vi "lab3.vi"() -> ()   [LabVIEW 2018]
uses:
  <vilib>/Utility/file.llb/Write Delimited Spreadsheet (DBL).vi
panel:
  out "unsigned byte array 2":u8[](array[numeric])
  out "Xincr":string
  out "Yoff":string
  out "Ymult":string
  out "error out 3":errorcluster
  in  "error in (no error) 4":errorcluster
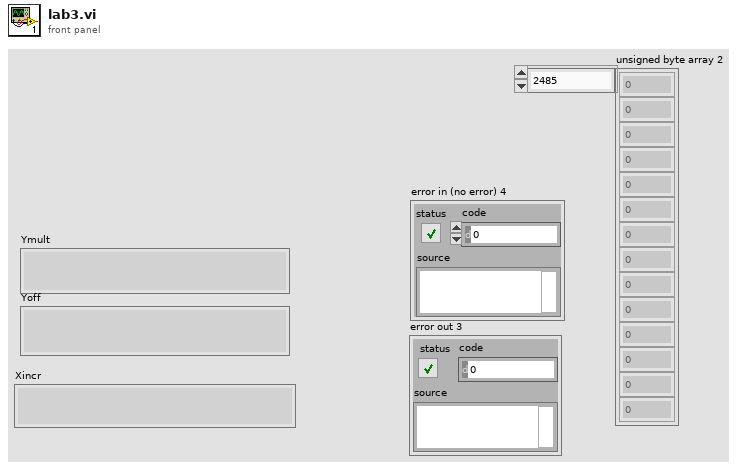
[diagram p1: front panel]
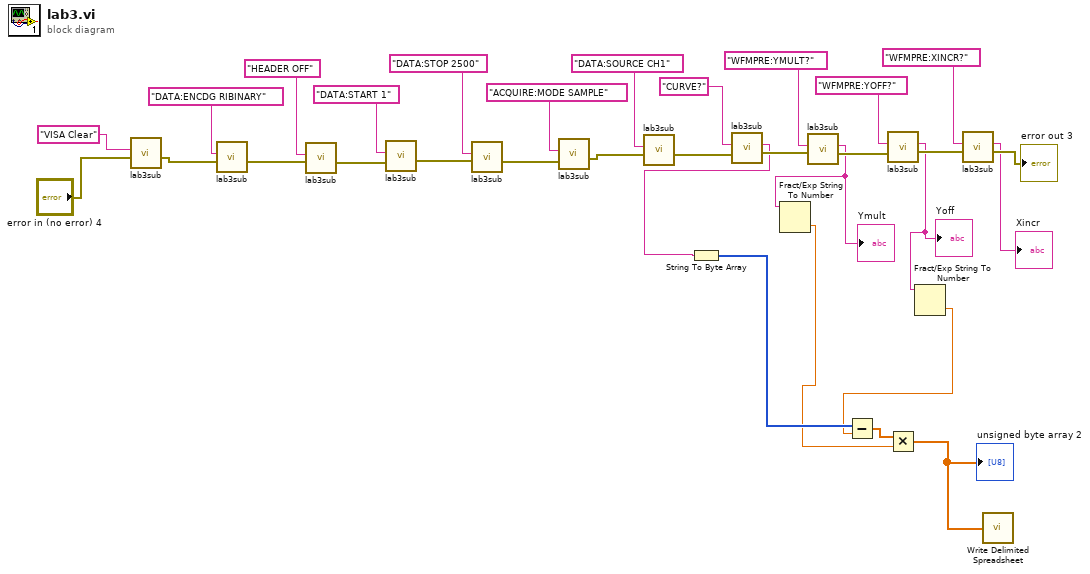
[diagram p0: block diagram]
diagram:
  n1 = call "lab3sub.vi"("error in (no error)"="error in (no error) 4", "write buffer"="VISA Clear") -> ("error out 2"=w21:errorcluster)  [unwired: 8 in, 1 out]
  n2 = call "lab3sub.vi"("error in (no error)"=w21, "write buffer"="DATA:ENCDG RIBINARY") -> ("error out 2"=w20:errorcluster)  [unwired: 8 in, 1 out]
  n3 = call "lab3sub.vi"("error in (no error)"=w20, "write buffer"="HEADER OFF") -> ("error out 2"=w19:errorcluster)  [unwired: 8 in, 1 out]
  n4 = call "lab3sub.vi"("error in (no error)"=w19, "write buffer"="DATA:START 1") -> ("error out 2"=w17:errorcluster)  [unwired: 8 in, 1 out]
  n5 = call "lab3sub.vi"("error in (no error)"=w17, "write buffer"="DATA:STOP 2500") -> ("error out 2"=w16:errorcluster)  [unwired: 8 in, 1 out]
  n6 = call "lab3sub.vi"("error in (no error)"=w16, "write buffer"="ACQUIRE:MODE SAMPLE") -> ("error out 2"=w15:errorcluster)  [unwired: 8 in, 1 out]
  n7 = call "lab3sub.vi"("error in (no error)"=w15, "write buffer"="DATA:SOURCE CH1") -> ("error out 2"=w14:errorcluster)  [unwired: 8 in, 1 out]
  n8 = call "lab3sub.vi"("error in (no error)"=w14, "write buffer"="CURVE?") -> ("error out 2"=w13:errorcluster, "read buffer"=w8:string)  [unwired: 8 in]
  n9 = String To Byte Array(string=w8) -> (unsigned byte array=w7:u8[])
  n10 = call "lab3sub.vi"("error in (no error)"=w13, "write buffer"="WFMPRE:YMULT?") -> ("error out 2"=w12:errorcluster, "read buffer"=w4:string)  [unwired: 8 in]
  "Ymult" <- w4
  n11 = Fract/Exp String To Number(string=w4) -> (number=w3:dbl)  [unwired: 3 in, 1 out]
  n12 = call "lab3sub.vi"("error in (no error)"=w12, "write buffer"="WFMPRE:YOFF?") -> ("error out 2"=w11:errorcluster, "read buffer"=w2:string)  [unwired: 8 in]
  "Yoff" <- w2
  n13 = Fract/Exp String To Number(string=w2) -> (number=w1:dbl)  [unwired: 3 in, 1 out]
  n14 = Subtract(x=w7, y=w1) -> (x-y=w6:dbl[])
  n15 = Multiply(x=w6, y=w3) -> (x*y=w5:dbl[])
  "unsigned byte array 2" <- w5
  n16 = call "lab3sub.vi"("error in (no error)"=w11, "write buffer"="WFMPRE:XINCR?") -> ("error out 2"=→"error out 3":errorcluster, "read buffer"=→"Xincr":string)  [unwired: 8 in]
  n17 = call-poly <vilib>:"Write Delimited Spreadsheet.vi"("1D data"=w5) -> ()  [unwired: 13 in, 2 out]
